vi "DO Command_TS.vi"(8 "error in (no error)":errorcluster, 10 "DO Command":bool[](array[boolean])) -> (0 "error out":errorcluster, 3 "VISA Refnum out":refnum<visa-resource-name>)   [LabVIEW 2022 SP3]
uses:
  <vilib>/Instr/_visa.llb/VISA Flush IO Buffer Mask.ctl
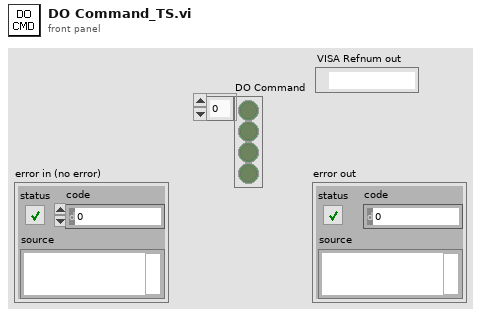
[diagram p1: front panel]
types:
  T1 = typedef "VISA Flush IO Buffer Mask.ctl" = u16
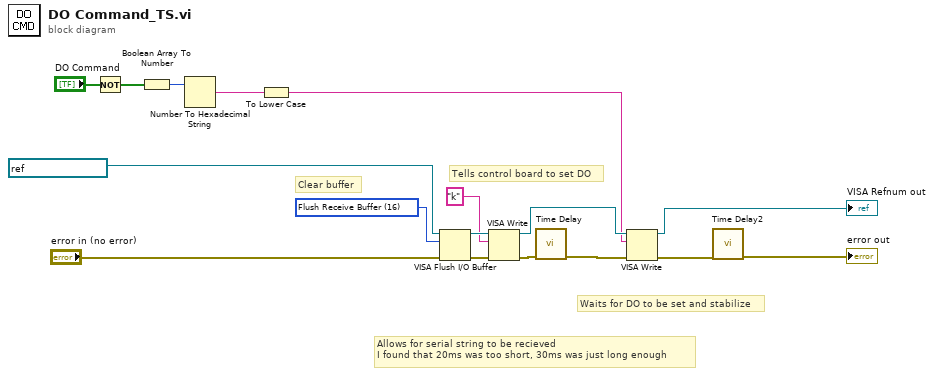
[diagram p0: block diagram]
diagram:
  w13 = T1 16 items=["Flush Receive Buffer"=16, "Write Transmit Buffer to Device"=32, "Flush Receive Buffer (No I/O)"=64, "Flush Transmit Buffer"=128] ("Mask")
  # "Waits for DO to be set and stabilize"
  # "Clear buffer"
  # "Allows for serial string to be recieved\nI found that 20ms was too short, 30ms was just long enough"
  # "Tells control board to set DO"
  n1 = Not(x="DO Command") -> (.not. x?=w4:bool[])
  n2 = Boolean Array To Number(Boolean array=w4) -> (number=w11:u32)
  n3 = Number To Hexadecimal String(2:w11) -> (0:w8:string)  [unwired: 1 in]
  n4 = To Lower Case(string=w8) -> (all lower case string=w5:string)
  n5 = VISA Flush I/O Buffer(VISA resource name=refnum<visa-resource-name> "ControlBoard", mask (16)=w13, error in (no error)="error in (no error)") -> (VISA resource name out=w15:refnum<visa-resource-name>, error out=w16:errorcluster)
  n6 = VISA Write(VISA resource name=w15, write buffer="k", error in (no error)=w16) -> (VISA resource name out=w6:refnum<visa-resource-name>, error out=w14:errorcluster)  [unwired: 1 out]
  n7 = call "Time Delay"("error in (no error)"=w14) -> ("error out"=w7:errorcluster)  [unwired: 10 in]
  n8 = VISA Write(VISA resource name=w6, write buffer=w5, error in (no error)=w7) -> (VISA resource name out=→"VISA Refnum out":refnum<visa-resource-name>, error out=w3:errorcluster)  [unwired: 1 out]
  n9 = call "Time Delay2"("error in (no error)"=w3) -> ("error out"=→"error out":errorcluster)  [unwired: 10 in]
